vi "Read currentState.vi"(8 "error in (no error)":errorcluster, 11 "WaitPassTactic in":refnum<class "WaitPassTactic.lvclass">) -> (0 "error out":errorcluster, 2 "Enum":T1, 3 "WaitPassTactic out":refnum<class "WaitPassTactic.lvclass">)   [LabVIEW 2023, in "WaitPassTactic.lvclass"]
uses:
  WaitPassTactic.lvclass
  WaitPassTactic_states_class/WaitPassTactic_states.ctl
  WaitPassTactic.lvclass/WaitPassTactic.ctl
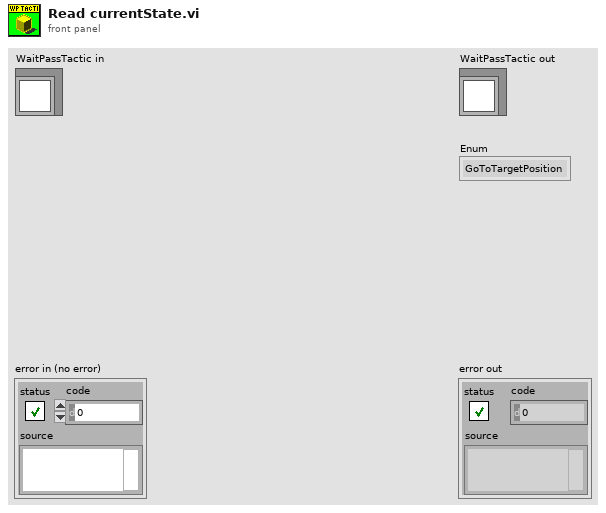
[diagram p1: front panel]
types:
  T1 = typedef "WaitPassTactic.lvclass/WaitPassTactic_states.ctl" = enum16{"GoToTargetPosition", "InterceptBall", "Exit"}
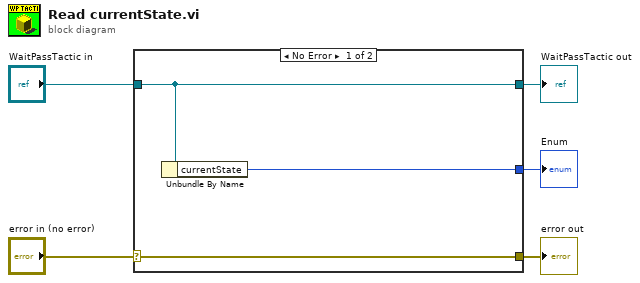
[diagram p0: block diagram]
diagram:
  n1 = case shown="No Error" "error in (no error)" {
    selector: "error in (no error)" -> [w8 w9]
    tunnel: [w8 w9] -> w4
    tunnel: [w7 w10] -> w2
    tunnel: "WaitPassTactic in" -> [w7 w10]
    tunnel: [w6 _] -> w1
    frame No Error {
      n2 = Unbundle By Name(w7) -> ("currentState"=w6:T1)
    }
    frame Error {
    }
  }
  "error out" <- w4
  "WaitPassTactic out" <- w2
  "Enum" <- w1
